vi "trafficlight_main_stateengine.vi"() -> ()   [LabVIEW 2022 SP3]
panel:
  in  "Standby Off":bool
  out "Ampel":cluster{"Red":bool, "Orange":bool, "Green":bool}
  in  "Stop":bool
  in  "Ampelzustände":T1(ring)
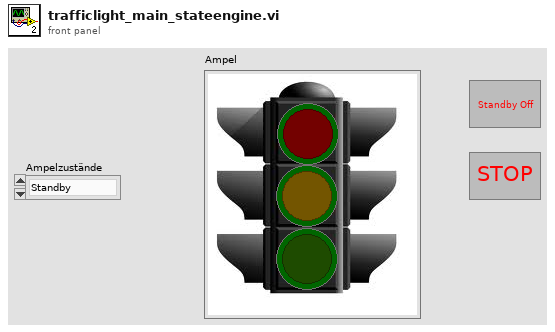
[diagram p1: front panel]
types:
  T1 = enum16{"Standby", "Red", "RedOrange", "Orange", "Green", "GreenBlinking"}
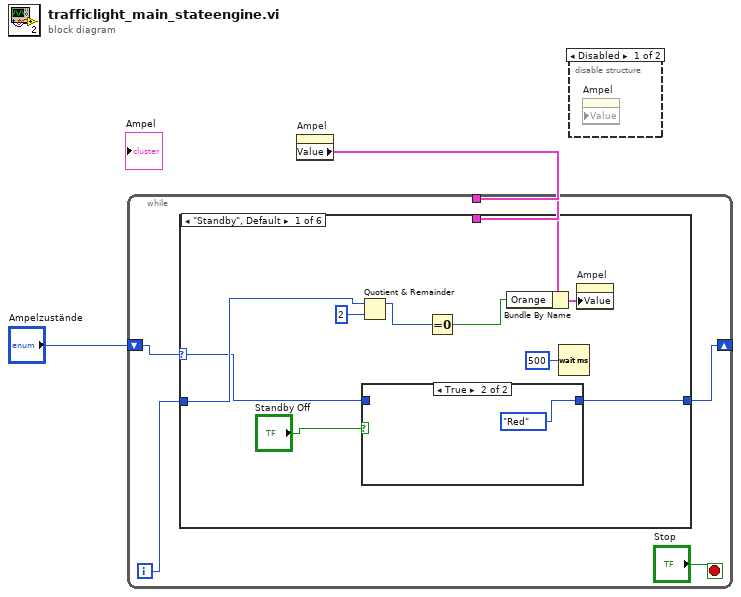
[diagram p0: block diagram]
diagram:
  n1 = property on="Ampel" class="Clust (strict)"() -> ("Value"=w1:cluster{"Red":bool, "Orange":bool, "Green":bool})  [unwired: 2 in, 2 out]
  n2 = while {
    shift-right: [w3] -> _
    shift-left: "Ampelzustände" -> [w5]
    tunnel: w1 -> [w6]
    i -> [w4]
    stop <- "Stop" stop-if-true
    n3 = case shown="\"Standby\", Default" w5 {
      selector: w5 -> [w10 _ _ _ _ _]
      tunnel: w6 -> [w17 _ _ _ _ _]
      tunnel: w4 -> [w11 _ _ _ _ _]
      tunnel: [w8 _ _ _ _ _] -> w3
      frame "Standby", Default {
        n4 = Quotient & Remainder(x=w11, y=2) -> (x-y*floor(x/y)=w13:i32)  [unwired: 1 out]
        n5 = case shown="True" "Standby Off" {
          tunnel: w10 -> [w18 _]
          tunnel: [w18 T1."Red" ("Enum")] -> w8
          frame False {
          }
          frame True {
          }
        }
        n6 = Equal To 0?(x=w13) -> (x = 0?=w12:bool)
        n7 = Bundle By Name(cluster=w17, "Orange"=w12) -> (w16:cluster{"Red":bool, "Orange":bool, "Green":bool})
        n8 = Wait (ms)(milliseconds to wait=u32 500) -> ()  [unwired: 1 out]
        n9 = property on="Ampel" class="Clust (strict)"("Value"=w16) -> ()  [unwired: 2 in, 2 out]
      }
      frame "Red" {
      }
      frame "RedOrange" {
      }
      frame "Orange" {
      }
      frame "Green" {
      }
      frame "GreenBlinking" {
      }
    }
  }
  n10 = disable-structure shown="Disabled" {
    frame Disabled {
      n11 = property on="Ampel" class="Clust (strict)" props=["Value"]() -> ()  [unwired: 3 in, 2 out]
    }
    frame Enabled {
    }
  }
